vi "calc_C345flipinvert.vi"(11 "Input U8":u8) -> (3 "Output U8":u8)   [LabVIEW 2018]
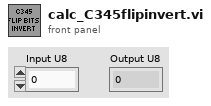
[diagram p1: front panel]
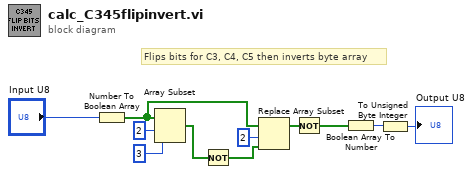
[diagram p0: block diagram]
diagram:
  # "Flips bits for C3, C4, C5 then inverts byte array"
  n1 = Number To Boolean Array(number="Input U8") -> (Boolean array=w5:bool[])
  n2 = Array Subset(array=w5, index=2, length=3) -> (w8:bool[])
  n3 = Not(x=w8) -> (.not. x?=w6:bool[])
  n4 = Replace Array Subset(array=w5, new element=w6, index=2) -> (w4:bool[])
  n5 = Not(x=w4) -> (.not. x?=w3:bool[])
  n6 = Boolean Array To Number(Boolean array=w3) -> (number=w2:u32)
  n7 = To Unsigned Byte Integer(number=w2) -> (unsigned 8bit integer=→"Output U8":u8)
